vi "Find StyleIndex by NumberingFormat.vi"(8 "error in":errorcluster, 10 "NumberingFormat Id":u32, 11 "Spreadsheet Doc in":refnum<k24>) -> (0 "error out":errorcluster, 2 "StyleIndex":u32, 3 "SpreadsheetDoc out":refnum<k24>)   [LabVIEW 2019, in "Open Xml.lvlib"]
uses:
  Open Xml.lvlib
  D:/git/Open-Xml-LabVIEW/Source/DocumentFormat.OpenXml.dll
  DocumentFormat.OpenXml.dll
  D:/git/Open-Xml-LabVIEW/Source/DocumentFormat.OpenXml.Framework.dll
  DocumentFormat.OpenXml.Framework.dll
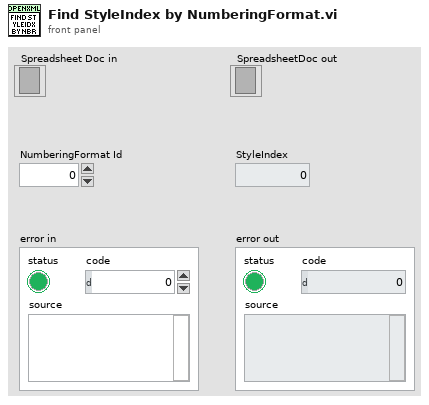
[diagram p1: front panel]
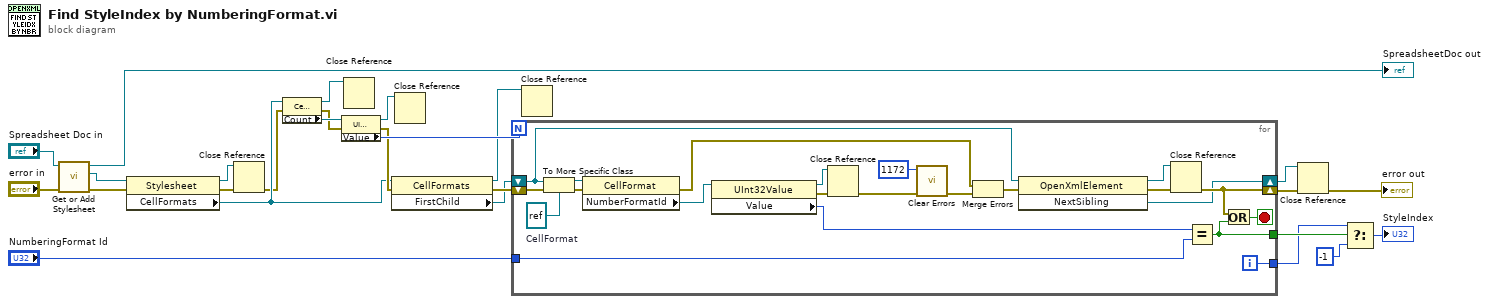
[diagram p0: block diagram]
diagram:
  n1 = call "Get or Add Stylesheet.vi"("error in"="error in", "SpreadsheetDoc in"="Spreadsheet Doc in") -> ("error out"=w25:errorcluster, "Stylesheet"=w23:refnum<k24>, "SpreadsheetDoc out"=→"SpreadsheetDoc out":refnum<k24>)  [unwired: 7 in]
  n2 = property class="Stylesheet"(reference=w23, error in=w25) -> (reference out=w1:refnum<k24>, error out=w20:errorcluster, "CellFormats"=w13:refnum<k24>)
  n3 = Close Reference(reference=w1, error in (no error)=w20) -> (error out=w2:errorcluster)
  n4 = property class="CellFormats"(reference=w13, error in=w2) -> (reference out=w22:refnum<k24>, error out=w17:errorcluster, "Count"=w21:refnum<k24>)
  n5 = property class="UInt32Value"(reference=w21, error in=w17) -> (reference out=w15:refnum<k24>, error out=w16:errorcluster, "Value"=w18:u32)
  n6 = Close Reference(reference=w22) -> ()  [unwired: 1 in, 1 out]
  n7 = property class="CellFormats"(reference=w13, error in=w16) -> (reference out=w12:refnum<k24>, error out=w14:errorcluster, "FirstChild"=w11:refnum<k24>)
  n8 = Close Reference(reference=w15) -> ()  [unwired: 1 in, 1 out]
  n9 = for {
    N: w18 -> [_]
    tunnel: "NumberingFormat Id" -> [w43]
    tunnel: [w42] -> w9
    tunnel: [w38] -> w6
    shift-right: [w29] -> w10
    shift-left: w14 -> [w48]
    shift-right: [w27] -> w3
    shift-left: w11 -> [w30]
    i -> [w38]
    stop <- w40 stop-if-true
    w47 = refnum<k24> refnum  # CellFormat
    n10 = To More Specific Class(target class=w47, reference=w30, error in=w48) -> (specific class reference=w45:refnum<k24>, error out=w46:errorcluster)
    n11 = property class="CellFormat"(reference=w45, error in=w46) -> (error out=w37:errorcluster, "NumberFormatId"=w44:refnum<k24>)  [unwired: 1 out]
    n12 = property class="UInt32Value"(reference=w44) -> (reference out=w32:refnum<k24>, error out=w36:errorcluster, "Value"=w41:u32)  [unwired: 1 in]
    n13 = Close Reference(reference=w32, error in (no error)=w36) -> (error out=w33:errorcluster)
    n14 = call <vilib>:"Clear Errors.vi"("error in (no error)"=w33, "specific error code to clear (0: all)"=1172) -> ("error out"=w35:errorcluster)  [unwired: 4 in, 1 out]
    n15 = Merge Errors(w37, w35) -> (w39:errorcluster)
    n16 = invoke class="OpenXmlElement" method="NextSibling"(reference=w30, error in=w39) -> (reference out=w28:refnum<k24>, error out=w31:errorcluster, "NextSibling"=w27:refnum<k24>)  [unwired: 1 in]
    n17 = Close Reference(reference=w28, error in (no error)=w31) -> (error out=w29:errorcluster)
    n18 = Equal?(x=w41, y=w43) -> (x = y?=w42:bool)
    n19 = Or(x=w29, y=w42) -> (x .or. y?=w40:bool)
  }
  n20 = Close Reference(reference=w12) -> ()  [unwired: 1 in, 1 out]
  n21 = Close Reference(reference=w3, error in (no error)=w10) -> (error out=→"error out":errorcluster)
  n22 = Select(t=w6, s=w9, f=-1) -> (s? t:f=→"StyleIndex":i32)
